vi "Experiment 20.vi"() -> ()   [LabVIEW 2026]
doc: "Experiment 20\nThis experiment is like Experiment 18 but uses while loops instead of for loops."
uses:
  <vilib>/AdvancedString/1D String Array to Delimited String (string).vi
  <vilib>/Analysis/baseanly.llb/Mean (DBL).vi
  <vilib>/Analysis/NI_AALBase.lvlib
panel:
  out "No. Of Iterations As Block Of Text (easy to copy into Excel)":string
  out "No. Of Iterations Executed - Loop 8":i32
  out "Output - Loop 8":dbl[](array[numeric]) format="%.3f"
  out "No. Of Iterations Executed - Loop 7":i32
  out "Output - Loop 7":dbl[](array[numeric]) format="%.3f"
  out "No. Of Iterations Executed - Loop 6":i32
  out "Output - Loop 6":dbl[](array[numeric]) format="%.3f"
  out "No. Of Iterations Executed - Loop 5":i32
  out "Output - Loop 5":dbl[](array[numeric]) format="%.3f"
  out "No. Of Iterations Executed - Loop 4":i32
  out "Output - Loop 4":dbl[](array[numeric]) format="%.3f"
  out "No. Of Iterations Executed - Loop 3":i32
  out "Output - Loop 3":dbl[](array[numeric]) format="%.3f"
  out "Avg. No. Of Iterations Executed - All Loops":dbl format="%.1f"
  out "No. Of Iterations Executed - Loop 2":i32
  out "Output - Loop 2":dbl[](array[numeric]) format="%.3f"
  out "No. Of Iterations Executed - Loop 1":i32
  out "Output - Loop 1":dbl[](array[numeric]) format="%.3f"
  out "Stop VI?":bool
  # "Experiment 20"
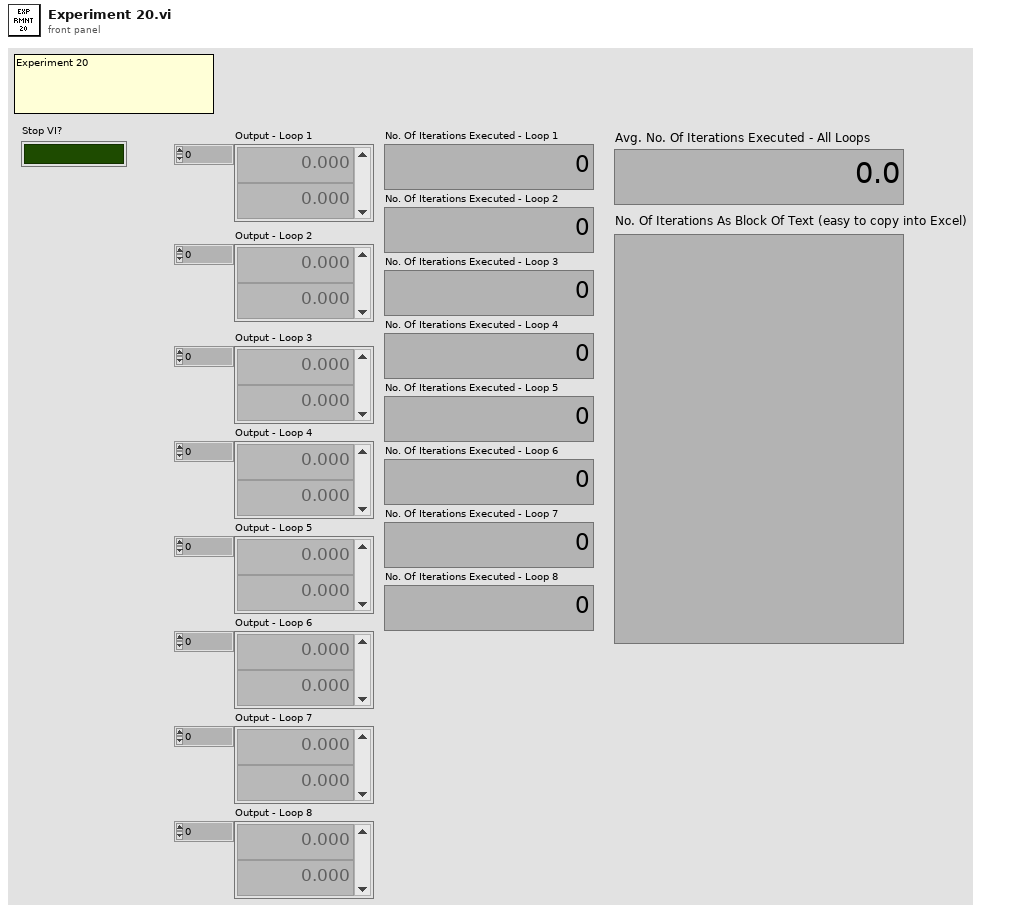
[diagram p1: front panel]
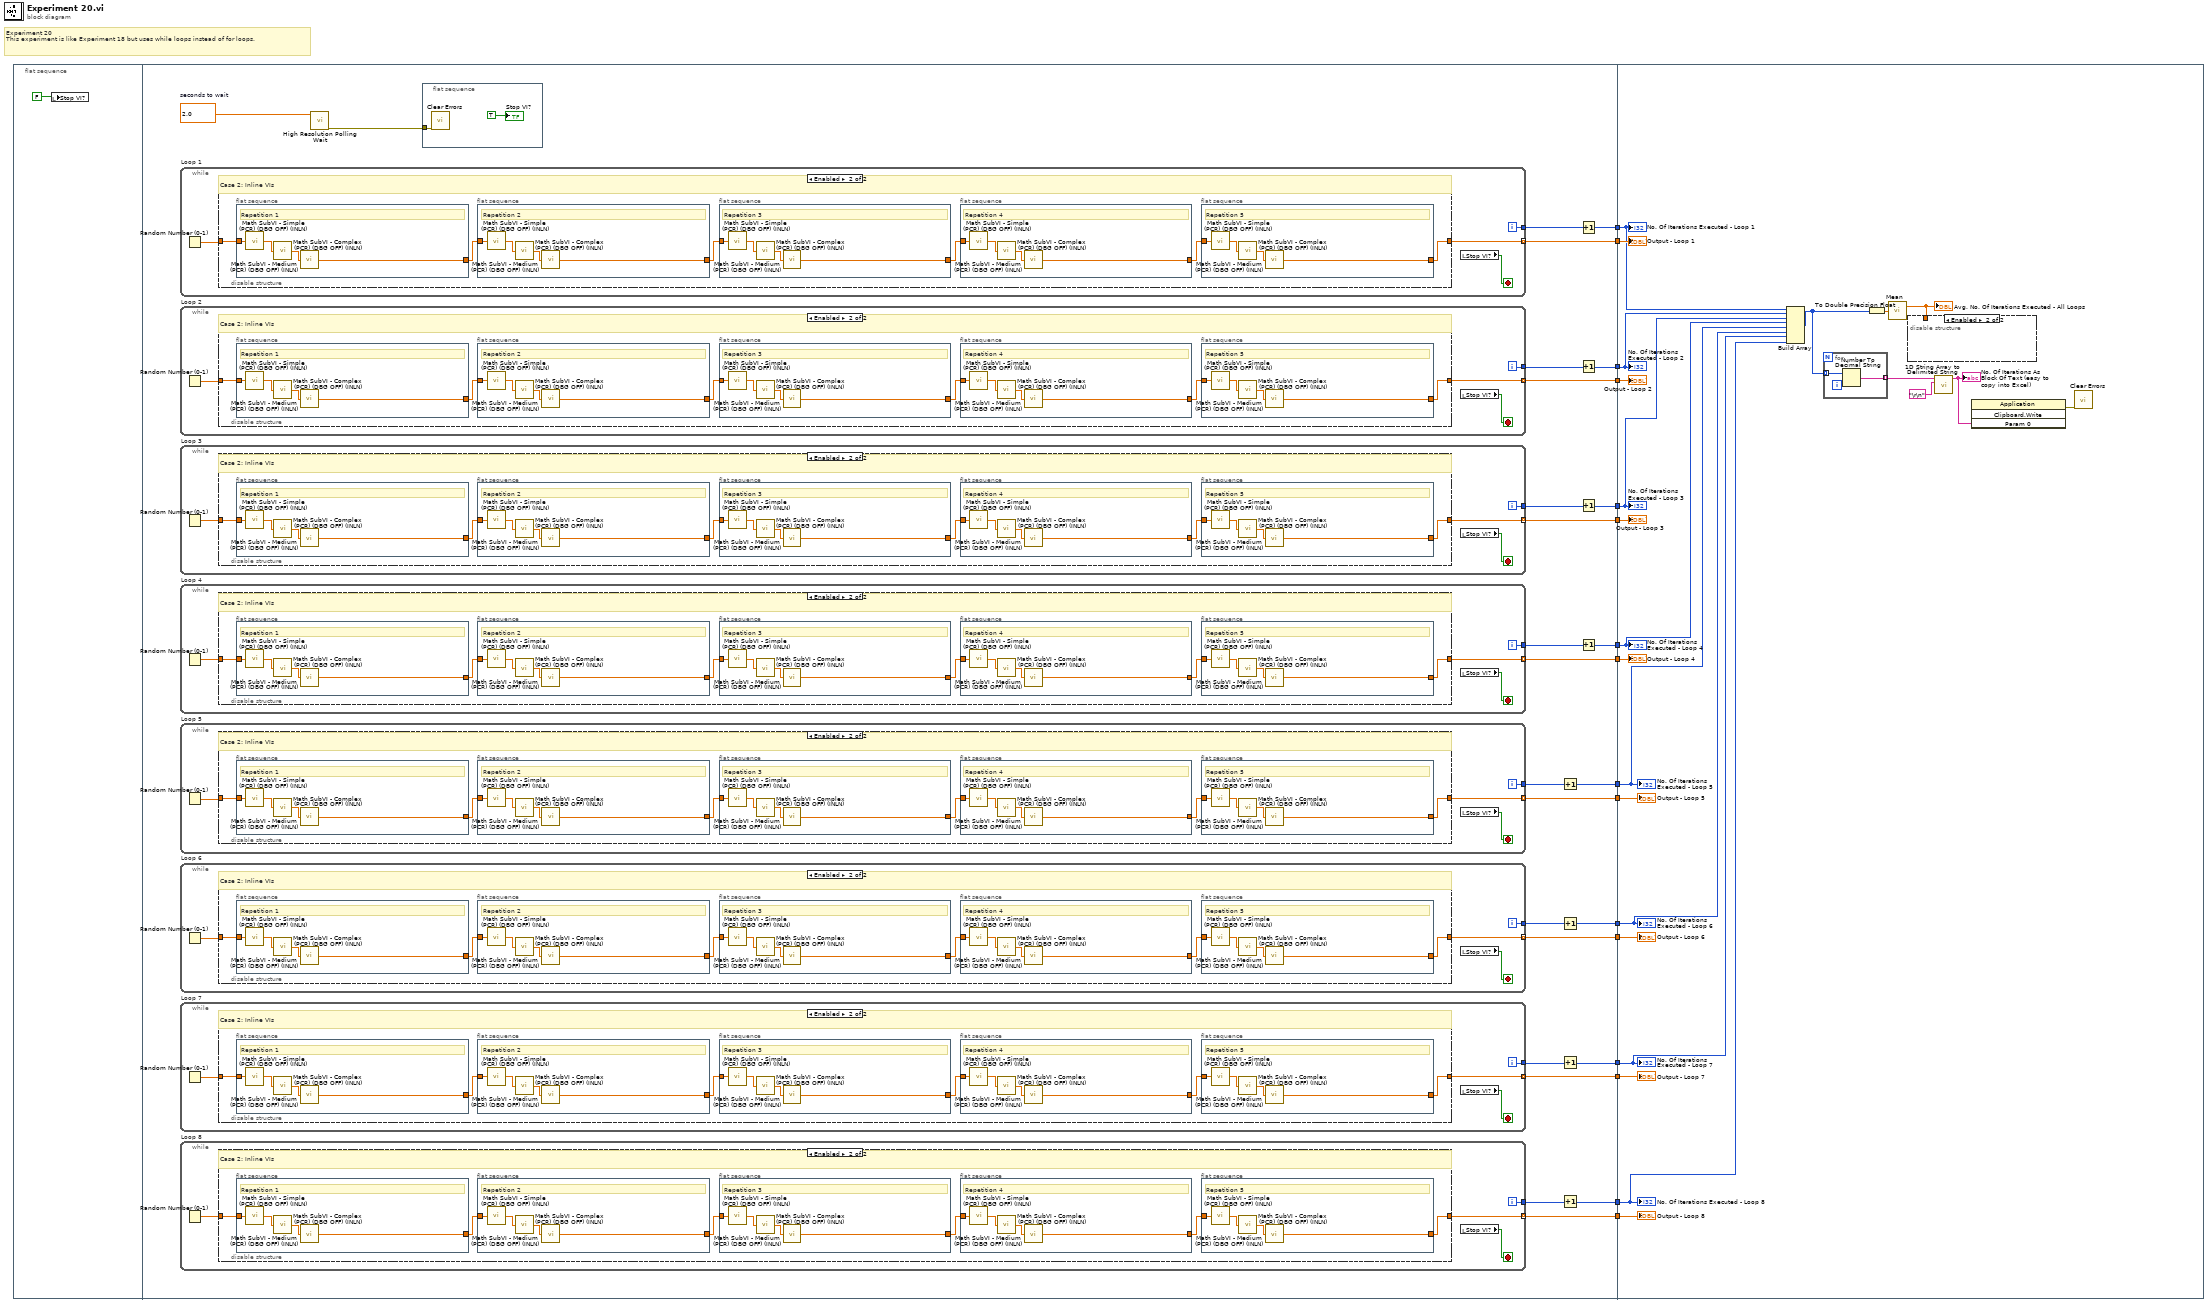
[diagram p0: block diagram]
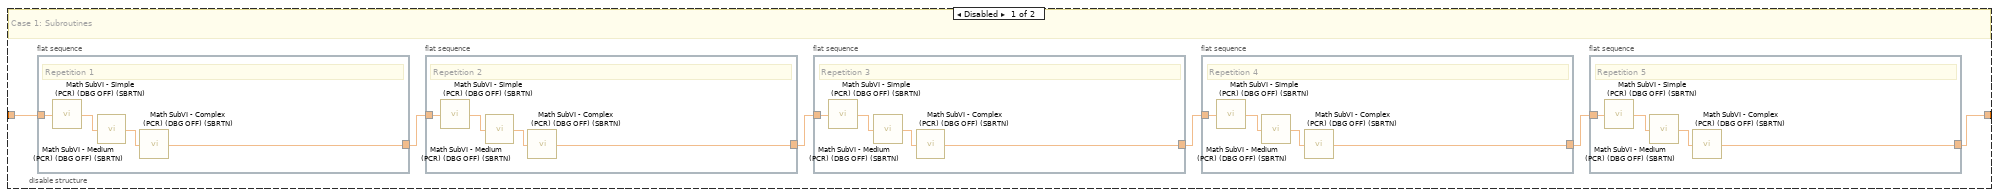
[diagram p2: hidden frame]
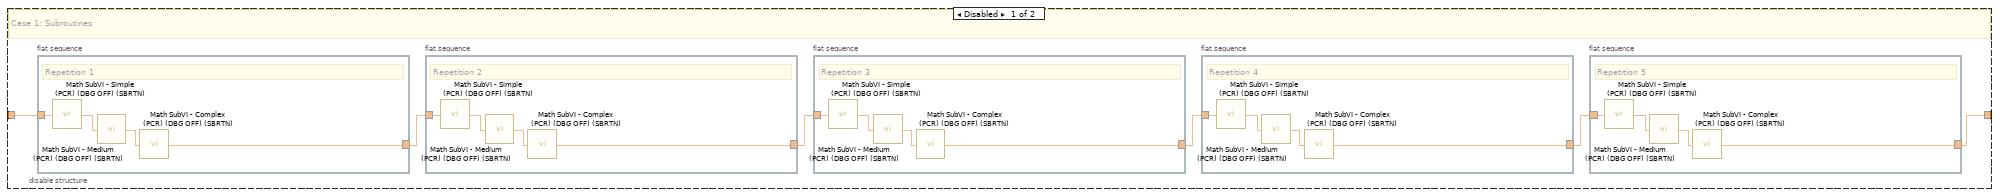
[diagram p3: hidden frame]
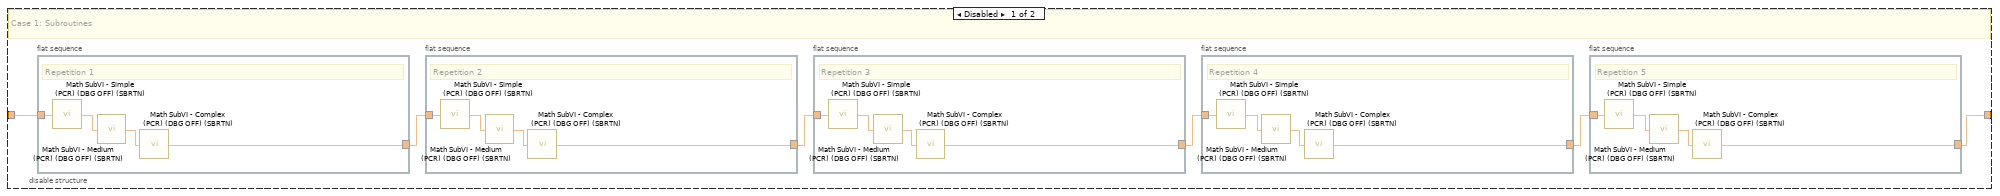
[diagram p4: hidden frame]
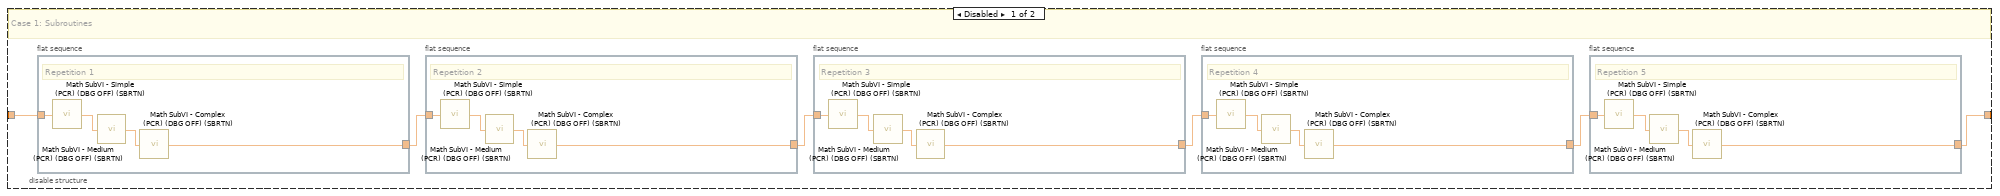
[diagram p5: hidden frame]
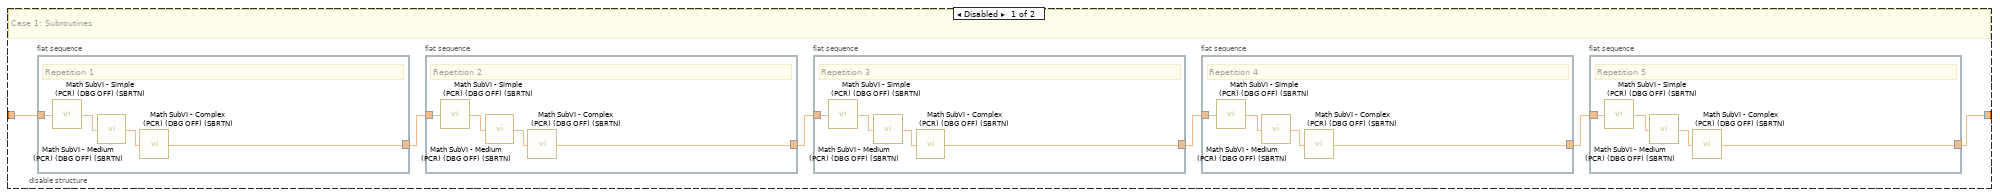
[diagram p6: hidden frame]
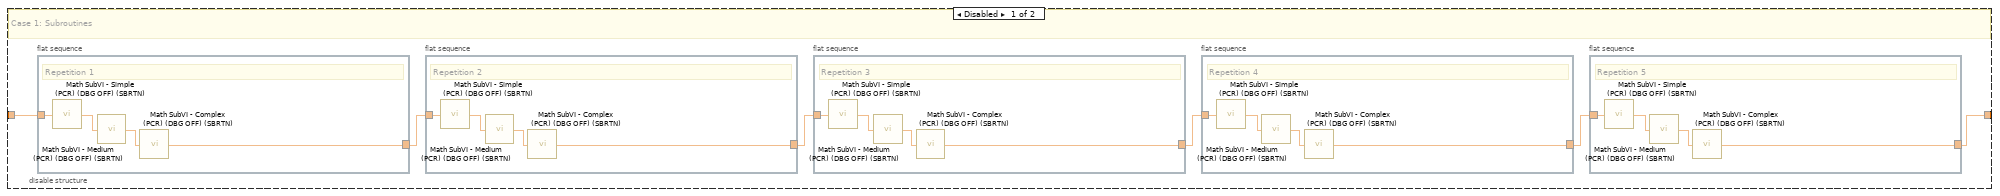
[diagram p7: hidden frame]
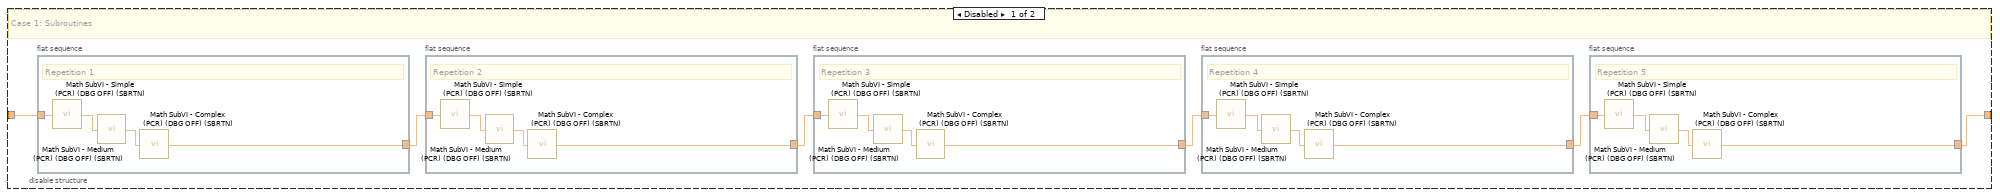
[diagram p8: hidden frame]
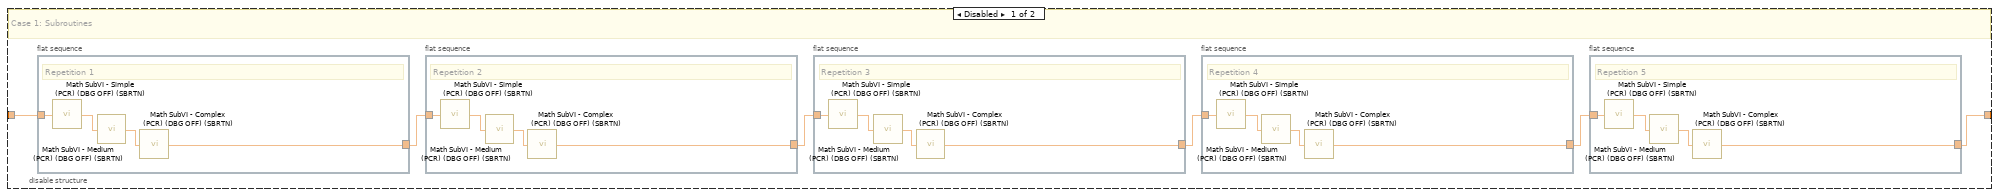
[diagram p9: hidden frame]
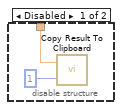
[diagram p10: hidden frame]
diagram:
  # "Experiment 20\nThis experiment is like Experiment 18 but uses while loops instead of for loops."
  n1 = flat-sequence {
    tunnel: [w41] -> w16
    tunnel: [w39] -> w15
    tunnel: [w38] -> w14
    tunnel: [w31] -> w13
    tunnel: [w37] -> w12
    tunnel: [w29] -> w11
    tunnel: [w27] -> w10
    tunnel: [w36] -> w9
    tunnel: [w25] -> w8
    tunnel: [w35] -> w7
    tunnel: [w23] -> w6
    tunnel: [w32] -> w5
    tunnel: [w21] -> w4
    tunnel: [w33] -> w3
    tunnel: [w18] -> w2
    tunnel: [w34] -> w1
    tunnel: w16 -> [w516]
    tunnel: w15 -> [w514]
    tunnel: w14 -> [w513]
    tunnel: w13 -> [w515]
    tunnel: w12 -> [w509]
    tunnel: w11 -> [w511]
    tunnel: w10 -> [w510]
    tunnel: w9 -> [w508]
    tunnel: w8 -> [w506]
    tunnel: w7 -> [w502]
    tunnel: w6 -> [w505]
    tunnel: w5 -> [w501]
    tunnel: w4 -> [w504]
    tunnel: w3 -> [w500]
    tunnel: w2 -> [w503]
    tunnel: w1 -> [w499]
    frame #0 {
      n2 = local write "Stop VI?"(FALSE) -> ()
    }
    frame #1 {
      w43 = 2.0  # seconds to wait
      n3 = while "Loop 1" {
        tunnel: [w437] -> w41 mode=indexing
        tunnel: [w438] -> w40
        i -> [w438]
        stop <- w439 stop-if-true
        n4 = Random Number (0-1)() -> (number: 0 to 1=w436:dbl)
        n5 = disable-structure shown="Enabled" {
          disable-tunnel: w436 -> [w445 w471]
          disable-tunnel: [w444 w466] -> w437
          frame Disabled {
            # "Case 1: Subroutines"
            n6 = flat-sequence {
              tunnel: w445 -> [w465]
              tunnel: [w462] -> w440
              frame #0 {
                # "Repetition 1"
                n7 = call "Math SubVI - Simple (PCR) (DBG OFF) (SBRTN).vi"("Input"=w465) -> ("Output"=w463:dbl)
                n8 = call "Math SubVI - Medium (PCR) (DBG OFF) (SBRTN).vi"("Input"=w463) -> ("Output"=w464:dbl)
                n9 = call "Math SubVI - Complex (PCR) (DBG OFF) (SBRTN).vi"("Input"=w464) -> ("Output"=w462:dbl)
              }
            }
            n10 = flat-sequence {
              tunnel: w440 -> [w461]
              tunnel: [w458] -> w443
              frame #0 {
                # "Repetition 2"
                n11 = call "Math SubVI - Simple (PCR) (DBG OFF) (SBRTN).vi"("Input"=w461) -> ("Output"=w459:dbl)
                n12 = call "Math SubVI - Medium (PCR) (DBG OFF) (SBRTN).vi"("Input"=w459) -> ("Output"=w460:dbl)
                n13 = call "Math SubVI - Complex (PCR) (DBG OFF) (SBRTN).vi"("Input"=w460) -> ("Output"=w458:dbl)
              }
            }
            n14 = flat-sequence {
              tunnel: w443 -> [w457]
              tunnel: [w454] -> w442
              frame #0 {
                # "Repetition 3"
                n15 = call "Math SubVI - Simple (PCR) (DBG OFF) (SBRTN).vi"("Input"=w457) -> ("Output"=w455:dbl)
                n16 = call "Math SubVI - Medium (PCR) (DBG OFF) (SBRTN).vi"("Input"=w455) -> ("Output"=w456:dbl)
                n17 = call "Math SubVI - Complex (PCR) (DBG OFF) (SBRTN).vi"("Input"=w456) -> ("Output"=w454:dbl)
              }
            }
            n18 = flat-sequence {
              tunnel: w442 -> [w453]
              tunnel: [w450] -> w441
              frame #0 {
                # "Repetition 4"
                n19 = call "Math SubVI - Simple (PCR) (DBG OFF) (SBRTN).vi"("Input"=w453) -> ("Output"=w451:dbl)
                n20 = call "Math SubVI - Medium (PCR) (DBG OFF) (SBRTN).vi"("Input"=w451) -> ("Output"=w452:dbl)
                n21 = call "Math SubVI - Complex (PCR) (DBG OFF) (SBRTN).vi"("Input"=w452) -> ("Output"=w450:dbl)
              }
            }
            n22 = flat-sequence {
              tunnel: w441 -> [w449]
              tunnel: [w446] -> w444
              frame #0 {
                # "Repetition 5"
                n23 = call "Math SubVI - Simple (PCR) (DBG OFF) (SBRTN).vi"("Input"=w449) -> ("Output"=w447:dbl)
                n24 = call "Math SubVI - Medium (PCR) (DBG OFF) (SBRTN).vi"("Input"=w447) -> ("Output"=w448:dbl)
                n25 = call "Math SubVI - Complex (PCR) (DBG OFF) (SBRTN).vi"("Input"=w448) -> ("Output"=w446:dbl)
              }
            }
          }
          frame Enabled {
            # "Case 2: Inline VIs"
            n26 = flat-sequence {
              tunnel: w471 -> [w491]
              tunnel: [w488] -> w470
              frame #0 {
                # "Repetition 1"
                n27 = call "Math SubVI - Simple (PCR) (DBG OFF) (INLN).vi"("Input"=w491) -> ("Output"=w489:dbl)
                n28 = call "Math SubVI - Medium (PCR) (DBG OFF) (INLN).vi"("Input"=w489) -> ("Output"=w490:dbl)
                n29 = call "Math SubVI - Complex (PCR) (DBG OFF) (INLN).vi"("Input"=w490) -> ("Output"=w488:dbl)
              }
            }
            n30 = flat-sequence {
              tunnel: w470 -> [w487]
              tunnel: [w484] -> w469
              frame #0 {
                # "Repetition 2"
                n31 = call "Math SubVI - Simple (PCR) (DBG OFF) (INLN).vi"("Input"=w487) -> ("Output"=w485:dbl)
                n32 = call "Math SubVI - Medium (PCR) (DBG OFF) (INLN).vi"("Input"=w485) -> ("Output"=w486:dbl)
                n33 = call "Math SubVI - Complex (PCR) (DBG OFF) (INLN).vi"("Input"=w486) -> ("Output"=w484:dbl)
              }
            }
            n34 = flat-sequence {
              tunnel: w469 -> [w483]
              tunnel: [w480] -> w468
              frame #0 {
                # "Repetition 3"
                n35 = call "Math SubVI - Simple (PCR) (DBG OFF) (INLN).vi"("Input"=w483) -> ("Output"=w481:dbl)
                n36 = call "Math SubVI - Medium (PCR) (DBG OFF) (INLN).vi"("Input"=w481) -> ("Output"=w482:dbl)
                n37 = call "Math SubVI - Complex (PCR) (DBG OFF) (INLN).vi"("Input"=w482) -> ("Output"=w480:dbl)
              }
            }
            n38 = flat-sequence {
              tunnel: w468 -> [w479]
              tunnel: [w476] -> w467
              frame #0 {
                # "Repetition 4"
                n39 = call "Math SubVI - Simple (PCR) (DBG OFF) (INLN).vi"("Input"=w479) -> ("Output"=w477:dbl)
                n40 = call "Math SubVI - Medium (PCR) (DBG OFF) (INLN).vi"("Input"=w477) -> ("Output"=w478:dbl)
                n41 = call "Math SubVI - Complex (PCR) (DBG OFF) (INLN).vi"("Input"=w478) -> ("Output"=w476:dbl)
              }
            }
            n42 = flat-sequence {
              tunnel: w467 -> [w475]
              tunnel: [w472] -> w466
              frame #0 {
                # "Repetition 5"
                n43 = call "Math SubVI - Simple (PCR) (DBG OFF) (INLN).vi"("Input"=w475) -> ("Output"=w473:dbl)
                n44 = call "Math SubVI - Medium (PCR) (DBG OFF) (INLN).vi"("Input"=w473) -> ("Output"=w474:dbl)
                n45 = call "Math SubVI - Complex (PCR) (DBG OFF) (INLN).vi"("Input"=w474) -> ("Output"=w472:dbl)
              }
            }
          }
        }
        n46 = local read "Stop VI?"() -> (w439:bool)
      }
      n47 = while "Loop 2" {
        tunnel: [w381] -> w31 mode=indexing
        tunnel: [w382] -> w30
        i -> [w382]
        stop <- w383 stop-if-true
        n48 = Random Number (0-1)() -> (number: 0 to 1=w380:dbl)
        n49 = disable-structure shown="Enabled" {
          disable-tunnel: w380 -> [w389 w415]
          disable-tunnel: [w388 w410] -> w381
          frame Disabled {
            # "Case 1: Subroutines"
            n50 = flat-sequence {
              tunnel: w389 -> [w409]
              tunnel: [w406] -> w384
              frame #0 {
                # "Repetition 1"
                n51 = call "Math SubVI - Simple (PCR) (DBG OFF) (SBRTN).vi"("Input"=w409) -> ("Output"=w407:dbl)
                n52 = call "Math SubVI - Medium (PCR) (DBG OFF) (SBRTN).vi"("Input"=w407) -> ("Output"=w408:dbl)
                n53 = call "Math SubVI - Complex (PCR) (DBG OFF) (SBRTN).vi"("Input"=w408) -> ("Output"=w406:dbl)
              }
            }
            n54 = flat-sequence {
              tunnel: w384 -> [w405]
              tunnel: [w402] -> w387
              frame #0 {
                # "Repetition 2"
                n55 = call "Math SubVI - Simple (PCR) (DBG OFF) (SBRTN).vi"("Input"=w405) -> ("Output"=w403:dbl)
                n56 = call "Math SubVI - Medium (PCR) (DBG OFF) (SBRTN).vi"("Input"=w403) -> ("Output"=w404:dbl)
                n57 = call "Math SubVI - Complex (PCR) (DBG OFF) (SBRTN).vi"("Input"=w404) -> ("Output"=w402:dbl)
              }
            }
            n58 = flat-sequence {
              tunnel: w387 -> [w401]
              tunnel: [w398] -> w386
              frame #0 {
                # "Repetition 3"
                n59 = call "Math SubVI - Simple (PCR) (DBG OFF) (SBRTN).vi"("Input"=w401) -> ("Output"=w399:dbl)
                n60 = call "Math SubVI - Medium (PCR) (DBG OFF) (SBRTN).vi"("Input"=w399) -> ("Output"=w400:dbl)
                n61 = call "Math SubVI - Complex (PCR) (DBG OFF) (SBRTN).vi"("Input"=w400) -> ("Output"=w398:dbl)
              }
            }
            n62 = flat-sequence {
              tunnel: w386 -> [w397]
              tunnel: [w394] -> w385
              frame #0 {
                # "Repetition 4"
                n63 = call "Math SubVI - Simple (PCR) (DBG OFF) (SBRTN).vi"("Input"=w397) -> ("Output"=w395:dbl)
                n64 = call "Math SubVI - Medium (PCR) (DBG OFF) (SBRTN).vi"("Input"=w395) -> ("Output"=w396:dbl)
                n65 = call "Math SubVI - Complex (PCR) (DBG OFF) (SBRTN).vi"("Input"=w396) -> ("Output"=w394:dbl)
              }
            }
            n66 = flat-sequence {
              tunnel: w385 -> [w393]
              tunnel: [w390] -> w388
              frame #0 {
                # "Repetition 5"
                n67 = call "Math SubVI - Simple (PCR) (DBG OFF) (SBRTN).vi"("Input"=w393) -> ("Output"=w391:dbl)
                n68 = call "Math SubVI - Medium (PCR) (DBG OFF) (SBRTN).vi"("Input"=w391) -> ("Output"=w392:dbl)
                n69 = call "Math SubVI - Complex (PCR) (DBG OFF) (SBRTN).vi"("Input"=w392) -> ("Output"=w390:dbl)
              }
            }
          }
          frame Enabled {
            # "Case 2: Inline VIs"
            n70 = flat-sequence {
              tunnel: w415 -> [w435]
              tunnel: [w432] -> w414
              frame #0 {
                # "Repetition 1"
                n71 = call "Math SubVI - Simple (PCR) (DBG OFF) (INLN).vi"("Input"=w435) -> ("Output"=w433:dbl)
                n72 = call "Math SubVI - Medium (PCR) (DBG OFF) (INLN).vi"("Input"=w433) -> ("Output"=w434:dbl)
                n73 = call "Math SubVI - Complex (PCR) (DBG OFF) (INLN).vi"("Input"=w434) -> ("Output"=w432:dbl)
              }
            }
            n74 = flat-sequence {
              tunnel: w414 -> [w431]
              tunnel: [w428] -> w413
              frame #0 {
                # "Repetition 2"
                n75 = call "Math SubVI - Simple (PCR) (DBG OFF) (INLN).vi"("Input"=w431) -> ("Output"=w429:dbl)
                n76 = call "Math SubVI - Medium (PCR) (DBG OFF) (INLN).vi"("Input"=w429) -> ("Output"=w430:dbl)
                n77 = call "Math SubVI - Complex (PCR) (DBG OFF) (INLN).vi"("Input"=w430) -> ("Output"=w428:dbl)
              }
            }
            n78 = flat-sequence {
              tunnel: w413 -> [w427]
              tunnel: [w424] -> w412
              frame #0 {
                # "Repetition 3"
                n79 = call "Math SubVI - Simple (PCR) (DBG OFF) (INLN).vi"("Input"=w427) -> ("Output"=w425:dbl)
                n80 = call "Math SubVI - Medium (PCR) (DBG OFF) (INLN).vi"("Input"=w425) -> ("Output"=w426:dbl)
                n81 = call "Math SubVI - Complex (PCR) (DBG OFF) (INLN).vi"("Input"=w426) -> ("Output"=w424:dbl)
              }
            }
            n82 = flat-sequence {
              tunnel: w412 -> [w423]
              tunnel: [w420] -> w411
              frame #0 {
                # "Repetition 4"
                n83 = call "Math SubVI - Simple (PCR) (DBG OFF) (INLN).vi"("Input"=w423) -> ("Output"=w421:dbl)
                n84 = call "Math SubVI - Medium (PCR) (DBG OFF) (INLN).vi"("Input"=w421) -> ("Output"=w422:dbl)
                n85 = call "Math SubVI - Complex (PCR) (DBG OFF) (INLN).vi"("Input"=w422) -> ("Output"=w420:dbl)
              }
            }
            n86 = flat-sequence {
              tunnel: w411 -> [w419]
              tunnel: [w416] -> w410
              frame #0 {
                # "Repetition 5"
                n87 = call "Math SubVI - Simple (PCR) (DBG OFF) (INLN).vi"("Input"=w419) -> ("Output"=w417:dbl)
                n88 = call "Math SubVI - Medium (PCR) (DBG OFF) (INLN).vi"("Input"=w417) -> ("Output"=w418:dbl)
                n89 = call "Math SubVI - Complex (PCR) (DBG OFF) (INLN).vi"("Input"=w418) -> ("Output"=w416:dbl)
              }
            }
          }
        }
        n90 = local read "Stop VI?"() -> (w383:bool)
      }
      n91 = while "Loop 3" {
        tunnel: [w325] -> w29 mode=indexing
        tunnel: [w326] -> w28
        i -> [w326]
        stop <- w327 stop-if-true
        n92 = Random Number (0-1)() -> (number: 0 to 1=w324:dbl)
        n93 = disable-structure shown="Enabled" {
          disable-tunnel: w324 -> [w333 w359]
          disable-tunnel: [w332 w354] -> w325
          frame Disabled {
            # "Case 1: Subroutines"
            n94 = flat-sequence {
              tunnel: w333 -> [w353]
              tunnel: [w350] -> w328
              frame #0 {
                # "Repetition 1"
                n95 = call "Math SubVI - Simple (PCR) (DBG OFF) (SBRTN).vi"("Input"=w353) -> ("Output"=w351:dbl)
                n96 = call "Math SubVI - Medium (PCR) (DBG OFF) (SBRTN).vi"("Input"=w351) -> ("Output"=w352:dbl)
                n97 = call "Math SubVI - Complex (PCR) (DBG OFF) (SBRTN).vi"("Input"=w352) -> ("Output"=w350:dbl)
              }
            }
            n98 = flat-sequence {
              tunnel: w328 -> [w349]
              tunnel: [w346] -> w331
              frame #0 {
                # "Repetition 2"
                n99 = call "Math SubVI - Simple (PCR) (DBG OFF) (SBRTN).vi"("Input"=w349) -> ("Output"=w347:dbl)
                n100 = call "Math SubVI - Medium (PCR) (DBG OFF) (SBRTN).vi"("Input"=w347) -> ("Output"=w348:dbl)
                n101 = call "Math SubVI - Complex (PCR) (DBG OFF) (SBRTN).vi"("Input"=w348) -> ("Output"=w346:dbl)
              }
            }
            n102 = flat-sequence {
              tunnel: w331 -> [w345]
              tunnel: [w342] -> w330
              frame #0 {
                # "Repetition 3"
                n103 = call "Math SubVI - Simple (PCR) (DBG OFF) (SBRTN).vi"("Input"=w345) -> ("Output"=w343:dbl)
                n104 = call "Math SubVI - Medium (PCR) (DBG OFF) (SBRTN).vi"("Input"=w343) -> ("Output"=w344:dbl)
                n105 = call "Math SubVI - Complex (PCR) (DBG OFF) (SBRTN).vi"("Input"=w344) -> ("Output"=w342:dbl)
              }
            }
            n106 = flat-sequence {
              tunnel: w330 -> [w341]
              tunnel: [w338] -> w329
              frame #0 {
                # "Repetition 4"
                n107 = call "Math SubVI - Simple (PCR) (DBG OFF) (SBRTN).vi"("Input"=w341) -> ("Output"=w339:dbl)
                n108 = call "Math SubVI - Medium (PCR) (DBG OFF) (SBRTN).vi"("Input"=w339) -> ("Output"=w340:dbl)
                n109 = call "Math SubVI - Complex (PCR) (DBG OFF) (SBRTN).vi"("Input"=w340) -> ("Output"=w338:dbl)
              }
            }
            n110 = flat-sequence {
              tunnel: w329 -> [w337]
              tunnel: [w334] -> w332
              frame #0 {
                # "Repetition 5"
                n111 = call "Math SubVI - Simple (PCR) (DBG OFF) (SBRTN).vi"("Input"=w337) -> ("Output"=w335:dbl)
                n112 = call "Math SubVI - Medium (PCR) (DBG OFF) (SBRTN).vi"("Input"=w335) -> ("Output"=w336:dbl)
                n113 = call "Math SubVI - Complex (PCR) (DBG OFF) (SBRTN).vi"("Input"=w336) -> ("Output"=w334:dbl)
              }
            }
          }
          frame Enabled {
            # "Case 2: Inline VIs"
            n114 = flat-sequence {
              tunnel: w359 -> [w379]
              tunnel: [w376] -> w358
              frame #0 {
                # "Repetition 1"
                n115 = call "Math SubVI - Simple (PCR) (DBG OFF) (INLN).vi"("Input"=w379) -> ("Output"=w377:dbl)
                n116 = call "Math SubVI - Medium (PCR) (DBG OFF) (INLN).vi"("Input"=w377) -> ("Output"=w378:dbl)
                n117 = call "Math SubVI - Complex (PCR) (DBG OFF) (INLN).vi"("Input"=w378) -> ("Output"=w376:dbl)
              }
            }
            n118 = flat-sequence {
              tunnel: w358 -> [w375]
              tunnel: [w372] -> w357
              frame #0 {
                # "Repetition 2"
                n119 = call "Math SubVI - Simple (PCR) (DBG OFF) (INLN).vi"("Input"=w375) -> ("Output"=w373:dbl)
                n120 = call "Math SubVI - Medium (PCR) (DBG OFF) (INLN).vi"("Input"=w373) -> ("Output"=w374:dbl)
                n121 = call "Math SubVI - Complex (PCR) (DBG OFF) (INLN).vi"("Input"=w374) -> ("Output"=w372:dbl)
              }
            }
            n122 = flat-sequence {
              tunnel: w357 -> [w371]
              tunnel: [w368] -> w356
              frame #0 {
                # "Repetition 3"
                n123 = call "Math SubVI - Simple (PCR) (DBG OFF) (INLN).vi"("Input"=w371) -> ("Output"=w369:dbl)
                n124 = call "Math SubVI - Medium (PCR) (DBG OFF) (INLN).vi"("Input"=w369) -> ("Output"=w370:dbl)
                n125 = call "Math SubVI - Complex (PCR) (DBG OFF) (INLN).vi"("Input"=w370) -> ("Output"=w368:dbl)
              }
            }
            n126 = flat-sequence {
              tunnel: w356 -> [w367]
              tunnel: [w364] -> w355
              frame #0 {
                # "Repetition 4"
                n127 = call "Math SubVI - Simple (PCR) (DBG OFF) (INLN).vi"("Input"=w367) -> ("Output"=w365:dbl)
                n128 = call "Math SubVI - Medium (PCR) (DBG OFF) (INLN).vi"("Input"=w365) -> ("Output"=w366:dbl)
                n129 = call "Math SubVI - Complex (PCR) (DBG OFF) (INLN).vi"("Input"=w366) -> ("Output"=w364:dbl)
              }
            }
            n130 = flat-sequence {
              tunnel: w355 -> [w363]
              tunnel: [w360] -> w354
              frame #0 {
                # "Repetition 5"
                n131 = call "Math SubVI - Simple (PCR) (DBG OFF) (INLN).vi"("Input"=w363) -> ("Output"=w361:dbl)
                n132 = call "Math SubVI - Medium (PCR) (DBG OFF) (INLN).vi"("Input"=w361) -> ("Output"=w362:dbl)
                n133 = call "Math SubVI - Complex (PCR) (DBG OFF) (INLN).vi"("Input"=w362) -> ("Output"=w360:dbl)
              }
            }
          }
        }
        n134 = local read "Stop VI?"() -> (w327:bool)
      }
      n135 = while "Loop 4" {
        tunnel: [w269] -> w27 mode=indexing
        tunnel: [w270] -> w26
        i -> [w270]
        stop <- w271 stop-if-true
        n136 = Random Number (0-1)() -> (number: 0 to 1=w268:dbl)
        n137 = disable-structure shown="Enabled" {
          disable-tunnel: w268 -> [w277 w303]
          disable-tunnel: [w276 w298] -> w269
          frame Disabled {
            # "Case 1: Subroutines"
            n138 = flat-sequence {
              tunnel: w277 -> [w297]
              tunnel: [w294] -> w272
              frame #0 {
                # "Repetition 1"
                n139 = call "Math SubVI - Simple (PCR) (DBG OFF) (SBRTN).vi"("Input"=w297) -> ("Output"=w295:dbl)
                n140 = call "Math SubVI - Medium (PCR) (DBG OFF) (SBRTN).vi"("Input"=w295) -> ("Output"=w296:dbl)
                n141 = call "Math SubVI - Complex (PCR) (DBG OFF) (SBRTN).vi"("Input"=w296) -> ("Output"=w294:dbl)
              }
            }
            n142 = flat-sequence {
              tunnel: w272 -> [w293]
              tunnel: [w290] -> w275
              frame #0 {
                # "Repetition 2"
                n143 = call "Math SubVI - Simple (PCR) (DBG OFF) (SBRTN).vi"("Input"=w293) -> ("Output"=w291:dbl)
                n144 = call "Math SubVI - Medium (PCR) (DBG OFF) (SBRTN).vi"("Input"=w291) -> ("Output"=w292:dbl)
                n145 = call "Math SubVI - Complex (PCR) (DBG OFF) (SBRTN).vi"("Input"=w292) -> ("Output"=w290:dbl)
              }
            }
            n146 = flat-sequence {
              tunnel: w275 -> [w289]
              tunnel: [w286] -> w274
              frame #0 {
                # "Repetition 3"
                n147 = call "Math SubVI - Simple (PCR) (DBG OFF) (SBRTN).vi"("Input"=w289) -> ("Output"=w287:dbl)
                n148 = call "Math SubVI - Medium (PCR) (DBG OFF) (SBRTN).vi"("Input"=w287) -> ("Output"=w288:dbl)
                n149 = call "Math SubVI - Complex (PCR) (DBG OFF) (SBRTN).vi"("Input"=w288) -> ("Output"=w286:dbl)
              }
            }
            n150 = flat-sequence {
              tunnel: w274 -> [w285]
              tunnel: [w282] -> w273
              frame #0 {
                # "Repetition 4"
                n151 = call "Math SubVI - Simple (PCR) (DBG OFF) (SBRTN).vi"("Input"=w285) -> ("Output"=w283:dbl)
                n152 = call "Math SubVI - Medium (PCR) (DBG OFF) (SBRTN).vi"("Input"=w283) -> ("Output"=w284:dbl)
                n153 = call "Math SubVI - Complex (PCR) (DBG OFF) (SBRTN).vi"("Input"=w284) -> ("Output"=w282:dbl)
              }
            }
            n154 = flat-sequence {
              tunnel: w273 -> [w281]
              tunnel: [w278] -> w276
              frame #0 {
                # "Repetition 5"
                n155 = call "Math SubVI - Simple (PCR) (DBG OFF) (SBRTN).vi"("Input"=w281) -> ("Output"=w279:dbl)
                n156 = call "Math SubVI - Medium (PCR) (DBG OFF) (SBRTN).vi"("Input"=w279) -> ("Output"=w280:dbl)
                n157 = call "Math SubVI - Complex (PCR) (DBG OFF) (SBRTN).vi"("Input"=w280) -> ("Output"=w278:dbl)
              }
            }
          }
          frame Enabled {
            # "Case 2: Inline VIs"
            n158 = flat-sequence {
              tunnel: w303 -> [w323]
              tunnel: [w320] -> w302
              frame #0 {
                # "Repetition 1"
                n159 = call "Math SubVI - Simple (PCR) (DBG OFF) (INLN).vi"("Input"=w323) -> ("Output"=w321:dbl)
                n160 = call "Math SubVI - Medium (PCR) (DBG OFF) (INLN).vi"("Input"=w321) -> ("Output"=w322:dbl)
                n161 = call "Math SubVI - Complex (PCR) (DBG OFF) (INLN).vi"("Input"=w322) -> ("Output"=w320:dbl)
              }
            }
            n162 = flat-sequence {
              tunnel: w302 -> [w319]
              tunnel: [w316] -> w301
              frame #0 {
                # "Repetition 2"
                n163 = call "Math SubVI - Simple (PCR) (DBG OFF) (INLN).vi"("Input"=w319) -> ("Output"=w317:dbl)
                n164 = call "Math SubVI - Medium (PCR) (DBG OFF) (INLN).vi"("Input"=w317) -> ("Output"=w318:dbl)
                n165 = call "Math SubVI - Complex (PCR) (DBG OFF) (INLN).vi"("Input"=w318) -> ("Output"=w316:dbl)
              }
            }
            n166 = flat-sequence {
              tunnel: w301 -> [w315]
              tunnel: [w312] -> w300
              frame #0 {
                # "Repetition 3"
                n167 = call "Math SubVI - Simple (PCR) (DBG OFF) (INLN).vi"("Input"=w315) -> ("Output"=w313:dbl)
                n168 = call "Math SubVI - Medium (PCR) (DBG OFF) (INLN).vi"("Input"=w313) -> ("Output"=w314:dbl)
                n169 = call "Math SubVI - Complex (PCR) (DBG OFF) (INLN).vi"("Input"=w314) -> ("Output"=w312:dbl)
              }
            }
            n170 = flat-sequence {
              tunnel: w300 -> [w311]
              tunnel: [w308] -> w299
              frame #0 {
                # "Repetition 4"
                n171 = call "Math SubVI - Simple (PCR) (DBG OFF) (INLN).vi"("Input"=w311) -> ("Output"=w309:dbl)
                n172 = call "Math SubVI - Medium (PCR) (DBG OFF) (INLN).vi"("Input"=w309) -> ("Output"=w310:dbl)
                n173 = call "Math SubVI - Complex (PCR) (DBG OFF) (INLN).vi"("Input"=w310) -> ("Output"=w308:dbl)
              }
            }
            n174 = flat-sequence {
              tunnel: w299 -> [w307]
              tunnel: [w304] -> w298
              frame #0 {
                # "Repetition 5"
                n175 = call "Math SubVI - Simple (PCR) (DBG OFF) (INLN).vi"("Input"=w307) -> ("Output"=w305:dbl)
                n176 = call "Math SubVI - Medium (PCR) (DBG OFF) (INLN).vi"("Input"=w305) -> ("Output"=w306:dbl)
                n177 = call "Math SubVI - Complex (PCR) (DBG OFF) (INLN).vi"("Input"=w306) -> ("Output"=w304:dbl)
              }
            }
          }
        }
        n178 = local read "Stop VI?"() -> (w271:bool)
      }
      n179 = while "Loop 5" {
        tunnel: [w213] -> w25 mode=indexing
        tunnel: [w214] -> w24
        i -> [w214]
        stop <- w215 stop-if-true
        n180 = Random Number (0-1)() -> (number: 0 to 1=w212:dbl)
        n181 = disable-structure shown="Enabled" {
          disable-tunnel: w212 -> [w221 w247]
          disable-tunnel: [w220 w242] -> w213
          frame Disabled {
            # "Case 1: Subroutines"
            n182 = flat-sequence {
              tunnel: w221 -> [w241]
              tunnel: [w238] -> w216
              frame #0 {
                # "Repetition 1"
                n183 = call "Math SubVI - Simple (PCR) (DBG OFF) (SBRTN).vi"("Input"=w241) -> ("Output"=w239:dbl)
                n184 = call "Math SubVI - Medium (PCR) (DBG OFF) (SBRTN).vi"("Input"=w239) -> ("Output"=w240:dbl)
                n185 = call "Math SubVI - Complex (PCR) (DBG OFF) (SBRTN).vi"("Input"=w240) -> ("Output"=w238:dbl)
              }
            }
            n186 = flat-sequence {
              tunnel: w216 -> [w237]
              tunnel: [w234] -> w219
              frame #0 {
                # "Repetition 2"
                n187 = call "Math SubVI - Simple (PCR) (DBG OFF) (SBRTN).vi"("Input"=w237) -> ("Output"=w235:dbl)
                n188 = call "Math SubVI - Medium (PCR) (DBG OFF) (SBRTN).vi"("Input"=w235) -> ("Output"=w236:dbl)
                n189 = call "Math SubVI - Complex (PCR) (DBG OFF) (SBRTN).vi"("Input"=w236) -> ("Output"=w234:dbl)
              }
            }
            n190 = flat-sequence {
              tunnel: w219 -> [w233]
              tunnel: [w230] -> w218
              frame #0 {
                # "Repetition 3"
                n191 = call "Math SubVI - Simple (PCR) (DBG OFF) (SBRTN).vi"("Input"=w233) -> ("Output"=w231:dbl)
                n192 = call "Math SubVI - Medium (PCR) (DBG OFF) (SBRTN).vi"("Input"=w231) -> ("Output"=w232:dbl)
                n193 = call "Math SubVI - Complex (PCR) (DBG OFF) (SBRTN).vi"("Input"=w232) -> ("Output"=w230:dbl)
              }
            }
            n194 = flat-sequence {
              tunnel: w218 -> [w229]
              tunnel: [w226] -> w217
              frame #0 {
                # "Repetition 4"
                n195 = call "Math SubVI - Simple (PCR) (DBG OFF) (SBRTN).vi"("Input"=w229) -> ("Output"=w227:dbl)
                n196 = call "Math SubVI - Medium (PCR) (DBG OFF) (SBRTN).vi"("Input"=w227) -> ("Output"=w228:dbl)
                n197 = call "Math SubVI - Complex (PCR) (DBG OFF) (SBRTN).vi"("Input"=w228) -> ("Output"=w226:dbl)
              }
            }
            n198 = flat-sequence {
              tunnel: w217 -> [w225]
              tunnel: [w222] -> w220
              frame #0 {
                # "Repetition 5"
                n199 = call "Math SubVI - Simple (PCR) (DBG OFF) (SBRTN).vi"("Input"=w225) -> ("Output"=w223:dbl)
                n200 = call "Math SubVI - Medium (PCR) (DBG OFF) (SBRTN).vi"("Input"=w223) -> ("Output"=w224:dbl)
                n201 = call "Math SubVI - Complex (PCR) (DBG OFF) (SBRTN).vi"("Input"=w224) -> ("Output"=w222:dbl)
              }
            }
          }
          frame Enabled {
            # "Case 2: Inline VIs"
            n202 = flat-sequence {
              tunnel: w247 -> [w267]
              tunnel: [w264] -> w246
              frame #0 {
                # "Repetition 1"
                n203 = call "Math SubVI - Simple (PCR) (DBG OFF) (INLN).vi"("Input"=w267) -> ("Output"=w265:dbl)
                n204 = call "Math SubVI - Medium (PCR) (DBG OFF) (INLN).vi"("Input"=w265) -> ("Output"=w266:dbl)
                n205 = call "Math SubVI - Complex (PCR) (DBG OFF) (INLN).vi"("Input"=w266) -> ("Output"=w264:dbl)
              }
            }
            n206 = flat-sequence {
              tunnel: w246 -> [w263]
              tunnel: [w260] -> w245
              frame #0 {
                # "Repetition 2"
                n207 = call "Math SubVI - Simple (PCR) (DBG OFF) (INLN).vi"("Input"=w263) -> ("Output"=w261:dbl)
                n208 = call "Math SubVI - Medium (PCR) (DBG OFF) (INLN).vi"("Input"=w261) -> ("Output"=w262:dbl)
                n209 = call "Math SubVI - Complex (PCR) (DBG OFF) (INLN).vi"("Input"=w262) -> ("Output"=w260:dbl)
              }
            }
            n210 = flat-sequence {
              tunnel: w245 -> [w259]
              tunnel: [w256] -> w244
              frame #0 {
                # "Repetition 3"
                n211 = call "Math SubVI - Simple (PCR) (DBG OFF) (INLN).vi"("Input"=w259) -> ("Output"=w257:dbl)
                n212 = call "Math SubVI - Medium (PCR) (DBG OFF) (INLN).vi"("Input"=w257) -> ("Output"=w258:dbl)
                n213 = call "Math SubVI - Complex (PCR) (DBG OFF) (INLN).vi"("Input"=w258) -> ("Output"=w256:dbl)
              }
            }
            n214 = flat-sequence {
              tunnel: w244 -> [w255]
              tunnel: [w252] -> w243
              frame #0 {
                # "Repetition 4"
                n215 = call "Math SubVI - Simple (PCR) (DBG OFF) (INLN).vi"("Input"=w255) -> ("Output"=w253:dbl)
                n216 = call "Math SubVI - Medium (PCR) (DBG OFF) (INLN).vi"("Input"=w253) -> ("Output"=w254:dbl)
                n217 = call "Math SubVI - Complex (PCR) (DBG OFF) (INLN).vi"("Input"=w254) -> ("Output"=w252:dbl)
              }
            }
            n218 = flat-sequence {
              tunnel: w243 -> [w251]
              tunnel: [w248] -> w242
              frame #0 {
                # "Repetition 5"
                n219 = call "Math SubVI - Simple (PCR) (DBG OFF) (INLN).vi"("Input"=w251) -> ("Output"=w249:dbl)
                n220 = call "Math SubVI - Medium (PCR) (DBG OFF) (INLN).vi"("Input"=w249) -> ("Output"=w250:dbl)
                n221 = call "Math SubVI - Complex (PCR) (DBG OFF) (INLN).vi"("Input"=w250) -> ("Output"=w248:dbl)
              }
            }
          }
        }
        n222 = local read "Stop VI?"() -> (w215:bool)
      }
      n223 = while "Loop 6" {
        tunnel: [w157] -> w23 mode=indexing
        tunnel: [w158] -> w22
        i -> [w158]
        stop <- w159 stop-if-true
        n224 = Random Number (0-1)() -> (number: 0 to 1=w156:dbl)
        n225 = disable-structure shown="Enabled" {
          disable-tunnel: w156 -> [w165 w191]
          disable-tunnel: [w164 w186] -> w157
          frame Disabled {
            # "Case 1: Subroutines"
            n226 = flat-sequence {
              tunnel: w165 -> [w185]
              tunnel: [w182] -> w160
              frame #0 {
                # "Repetition 1"
                n227 = call "Math SubVI - Simple (PCR) (DBG OFF) (SBRTN).vi"("Input"=w185) -> ("Output"=w183:dbl)
                n228 = call "Math SubVI - Medium (PCR) (DBG OFF) (SBRTN).vi"("Input"=w183) -> ("Output"=w184:dbl)
                n229 = call "Math SubVI - Complex (PCR) (DBG OFF) (SBRTN).vi"("Input"=w184) -> ("Output"=w182:dbl)
              }
            }
            n230 = flat-sequence {
              tunnel: w160 -> [w181]
              tunnel: [w178] -> w163
              frame #0 {
                # "Repetition 2"
                n231 = call "Math SubVI - Simple (PCR) (DBG OFF) (SBRTN).vi"("Input"=w181) -> ("Output"=w179:dbl)
                n232 = call "Math SubVI - Medium (PCR) (DBG OFF) (SBRTN).vi"("Input"=w179) -> ("Output"=w180:dbl)
                n233 = call "Math SubVI - Complex (PCR) (DBG OFF) (SBRTN).vi"("Input"=w180) -> ("Output"=w178:dbl)
              }
            }
            n234 = flat-sequence {
              tunnel: w163 -> [w177]
              tunnel: [w174] -> w162
              frame #0 {
                # "Repetition 3"
                n235 = call "Math SubVI - Simple (PCR) (DBG OFF) (SBRTN).vi"("Input"=w177) -> ("Output"=w175:dbl)
                n236 = call "Math SubVI - Medium (PCR) (DBG OFF) (SBRTN).vi"("Input"=w175) -> ("Output"=w176:dbl)
                n237 = call "Math SubVI - Complex (PCR) (DBG OFF) (SBRTN).vi"("Input"=w176) -> ("Output"=w174:dbl)
              }
            }
            n238 = flat-sequence {
              tunnel: w162 -> [w173]
              tunnel: [w170] -> w161
              frame #0 {
                # "Repetition 4"
                n239 = call "Math SubVI - Simple (PCR) (DBG OFF) (SBRTN).vi"("Input"=w173) -> ("Output"=w171:dbl)
                n240 = call "Math SubVI - Medium (PCR) (DBG OFF) (SBRTN).vi"("Input"=w171) -> ("Output"=w172:dbl)
                n241 = call "Math SubVI - Complex (PCR) (DBG OFF) (SBRTN).vi"("Input"=w172) -> ("Output"=w170:dbl)
              }
            }
            n242 = flat-sequence {
              tunnel: w161 -> [w169]
              tunnel: [w166] -> w164
              frame #0 {
                # "Repetition 5"
                n243 = call "Math SubVI - Simple (PCR) (DBG OFF) (SBRTN).vi"("Input"=w169) -> ("Output"=w167:dbl)
                n244 = call "Math SubVI - Medium (PCR) (DBG OFF) (SBRTN).vi"("Input"=w167) -> ("Output"=w168:dbl)
                n245 = call "Math SubVI - Complex (PCR) (DBG OFF) (SBRTN).vi"("Input"=w168) -> ("Output"=w166:dbl)
              }
            }
          }
          frame Enabled {
            # "Case 2: Inline VIs"
            n246 = flat-sequence {
              tunnel: w191 -> [w211]
              tunnel: [w208] -> w190
              frame #0 {
                # "Repetition 1"
                n247 = call "Math SubVI - Simple (PCR) (DBG OFF) (INLN).vi"("Input"=w211) -> ("Output"=w209:dbl)
                n248 = call "Math SubVI - Medium (PCR) (DBG OFF) (INLN).vi"("Input"=w209) -> ("Output"=w210:dbl)
                n249 = call "Math SubVI - Complex (PCR) (DBG OFF) (INLN).vi"("Input"=w210) -> ("Output"=w208:dbl)
              }
            }
            n250 = flat-sequence {
              tunnel: w190 -> [w207]
              tunnel: [w204] -> w189
              frame #0 {
                # "Repetition 2"
                n251 = call "Math SubVI - Simple (PCR) (DBG OFF) (INLN).vi"("Input"=w207) -> ("Output"=w205:dbl)
                n252 = call "Math SubVI - Medium (PCR) (DBG OFF) (INLN).vi"("Input"=w205) -> ("Output"=w206:dbl)
                n253 = call "Math SubVI - Complex (PCR) (DBG OFF) (INLN).vi"("Input"=w206) -> ("Output"=w204:dbl)
              }
            }
            n254 = flat-sequence {
              tunnel: w189 -> [w203]
              tunnel: [w200] -> w188
              frame #0 {
                # "Repetition 3"
                n255 = call "Math SubVI - Simple (PCR) (DBG OFF) (INLN).vi"("Input"=w203) -> ("Output"=w201:dbl)
                n256 = call "Math SubVI - Medium (PCR) (DBG OFF) (INLN).vi"("Input"=w201) -> ("Output"=w202:dbl)
                n257 = call "Math SubVI - Complex (PCR) (DBG OFF) (INLN).vi"("Input"=w202) -> ("Output"=w200:dbl)
              }
            }
            n258 = flat-sequence {
              tunnel: w188 -> [w199]
              tunnel: [w196] -> w187
              frame #0 {
                # "Repetition 4"
                n259 = call "Math SubVI - Simple (PCR) (DBG OFF) (INLN).vi"("Input"=w199) -> ("Output"=w197:dbl)
                n260 = call "Math SubVI - Medium (PCR) (DBG OFF) (INLN).vi"("Input"=w197) -> ("Output"=w198:dbl)
                n261 = call "Math SubVI - Complex (PCR) (DBG OFF) (INLN).vi"("Input"=w198) -> ("Output"=w196:dbl)
              }
            }
            n262 = flat-sequence {
              tunnel: w187 -> [w195]
              tunnel: [w192] -> w186
              frame #0 {
                # "Repetition 5"
                n263 = call "Math SubVI - Simple (PCR) (DBG OFF) (INLN).vi"("Input"=w195) -> ("Output"=w193:dbl)
                n264 = call "Math SubVI - Medium (PCR) (DBG OFF) (INLN).vi"("Input"=w193) -> ("Output"=w194:dbl)
                n265 = call "Math SubVI - Complex (PCR) (DBG OFF) (INLN).vi"("Input"=w194) -> ("Output"=w192:dbl)
              }
            }
          }
        }
        n266 = local read "Stop VI?"() -> (w159:bool)
      }
      n267 = while "Loop 7" {
        tunnel: [w101] -> w21 mode=indexing
        tunnel: [w102] -> w20
        i -> [w102]
        stop <- w103 stop-if-true
        n268 = Random Number (0-1)() -> (number: 0 to 1=w100:dbl)
        n269 = disable-structure shown="Enabled" {
          disable-tunnel: w100 -> [w109 w135]
          disable-tunnel: [w108 w130] -> w101
          frame Disabled {
            # "Case 1: Subroutines"
            n270 = flat-sequence {
              tunnel: w109 -> [w129]
              tunnel: [w126] -> w104
              frame #0 {
                # "Repetition 1"
                n271 = call "Math SubVI - Simple (PCR) (DBG OFF) (SBRTN).vi"("Input"=w129) -> ("Output"=w127:dbl)
                n272 = call "Math SubVI - Medium (PCR) (DBG OFF) (SBRTN).vi"("Input"=w127) -> ("Output"=w128:dbl)
                n273 = call "Math SubVI - Complex (PCR) (DBG OFF) (SBRTN).vi"("Input"=w128) -> ("Output"=w126:dbl)
              }
            }
            n274 = flat-sequence {
              tunnel: w104 -> [w125]
              tunnel: [w122] -> w107
              frame #0 {
                # "Repetition 2"
                n275 = call "Math SubVI - Simple (PCR) (DBG OFF) (SBRTN).vi"("Input"=w125) -> ("Output"=w123:dbl)
                n276 = call "Math SubVI - Medium (PCR) (DBG OFF) (SBRTN).vi"("Input"=w123) -> ("Output"=w124:dbl)
                n277 = call "Math SubVI - Complex (PCR) (DBG OFF) (SBRTN).vi"("Input"=w124) -> ("Output"=w122:dbl)
              }
            }
            n278 = flat-sequence {
              tunnel: w107 -> [w121]
              tunnel: [w118] -> w106
              frame #0 {
                # "Repetition 3"
                n279 = call "Math SubVI - Simple (PCR) (DBG OFF) (SBRTN).vi"("Input"=w121) -> ("Output"=w119:dbl)
                n280 = call "Math SubVI - Medium (PCR) (DBG OFF) (SBRTN).vi"("Input"=w119) -> ("Output"=w120:dbl)
                n281 = call "Math SubVI - Complex (PCR) (DBG OFF) (SBRTN).vi"("Input"=w120) -> ("Output"=w118:dbl)
              }
            }
            n282 = flat-sequence {
              tunnel: w106 -> [w117]
              tunnel: [w114] -> w105
              frame #0 {
                # "Repetition 4"
                n283 = call "Math SubVI - Simple (PCR) (DBG OFF) (SBRTN).vi"("Input"=w117) -> ("Output"=w115:dbl)
                n284 = call "Math SubVI - Medium (PCR) (DBG OFF) (SBRTN).vi"("Input"=w115) -> ("Output"=w116:dbl)
                n285 = call "Math SubVI - Complex (PCR) (DBG OFF) (SBRTN).vi"("Input"=w116) -> ("Output"=w114:dbl)
              }
            }
            n286 = flat-sequence {
              tunnel: w105 -> [w113]
              tunnel: [w110] -> w108
              frame #0 {
                # "Repetition 5"
                n287 = call "Math SubVI - Simple (PCR) (DBG OFF) (SBRTN).vi"("Input"=w113) -> ("Output"=w111:dbl)
                n288 = call "Math SubVI - Medium (PCR) (DBG OFF) (SBRTN).vi"("Input"=w111) -> ("Output"=w112:dbl)
                n289 = call "Math SubVI - Complex (PCR) (DBG OFF) (SBRTN).vi"("Input"=w112) -> ("Output"=w110:dbl)
              }
            }
          }
          frame Enabled {
            # "Case 2: Inline VIs"
            n290 = flat-sequence {
              tunnel: w135 -> [w155]
              tunnel: [w152] -> w134
              frame #0 {
                # "Repetition 1"
                n291 = call "Math SubVI - Simple (PCR) (DBG OFF) (INLN).vi"("Input"=w155) -> ("Output"=w153:dbl)
                n292 = call "Math SubVI - Medium (PCR) (DBG OFF) (INLN).vi"("Input"=w153) -> ("Output"=w154:dbl)
                n293 = call "Math SubVI - Complex (PCR) (DBG OFF) (INLN).vi"("Input"=w154) -> ("Output"=w152:dbl)
              }
            }
            n294 = flat-sequence {
              tunnel: w134 -> [w151]
              tunnel: [w148] -> w133
              frame #0 {
                # "Repetition 2"
                n295 = call "Math SubVI - Simple (PCR) (DBG OFF) (INLN).vi"("Input"=w151) -> ("Output"=w149:dbl)
                n296 = call "Math SubVI - Medium (PCR) (DBG OFF) (INLN).vi"("Input"=w149) -> ("Output"=w150:dbl)
                n297 = call "Math SubVI - Complex (PCR) (DBG OFF) (INLN).vi"("Input"=w150) -> ("Output"=w148:dbl)
              }
            }
            n298 = flat-sequence {
              tunnel: w133 -> [w147]
              tunnel: [w144] -> w132
              frame #0 {
                # "Repetition 3"
                n299 = call "Math SubVI - Simple (PCR) (DBG OFF) (INLN).vi"("Input"=w147) -> ("Output"=w145:dbl)
                n300 = call "Math SubVI - Medium (PCR) (DBG OFF) (INLN).vi"("Input"=w145) -> ("Output"=w146:dbl)
                n301 = call "Math SubVI - Complex (PCR) (DBG OFF) (INLN).vi"("Input"=w146) -> ("Output"=w144:dbl)
              }
            }
            n302 = flat-sequence {
              tunnel: w132 -> [w143]
              tunnel: [w140] -> w131
              frame #0 {
                # "Repetition 4"
                n303 = call "Math SubVI - Simple (PCR) (DBG OFF) (INLN).vi"("Input"=w143) -> ("Output"=w141:dbl)
                n304 = call "Math SubVI - Medium (PCR) (DBG OFF) (INLN).vi"("Input"=w141) -> ("Output"=w142:dbl)
                n305 = call "Math SubVI - Complex (PCR) (DBG OFF) (INLN).vi"("Input"=w142) -> ("Output"=w140:dbl)
              }
            }
            n306 = flat-sequence {
              tunnel: w131 -> [w139]
              tunnel: [w136] -> w130
              frame #0 {
                # "Repetition 5"
                n307 = call "Math SubVI - Simple (PCR) (DBG OFF) (INLN).vi"("Input"=w139) -> ("Output"=w137:dbl)
                n308 = call "Math SubVI - Medium (PCR) (DBG OFF) (INLN).vi"("Input"=w137) -> ("Output"=w138:dbl)
                n309 = call "Math SubVI - Complex (PCR) (DBG OFF) (INLN).vi"("Input"=w138) -> ("Output"=w136:dbl)
              }
            }
          }
        }
        n310 = local read "Stop VI?"() -> (w103:bool)
      }
      n311 = while "Loop 8" {
        tunnel: [w45] -> w18 mode=indexing
        tunnel: [w46] -> w19
        i -> [w46]
        stop <- w47 stop-if-true
        n312 = Random Number (0-1)() -> (number: 0 to 1=w44:dbl)
        n313 = disable-structure shown="Enabled" {
          disable-tunnel: w44 -> [w53 w79]
          disable-tunnel: [w52 w74] -> w45
          frame Disabled {
            # "Case 1: Subroutines"
            n314 = flat-sequence {
              tunnel: w53 -> [w73]
              tunnel: [w70] -> w48
              frame #0 {
                # "Repetition 1"
                n315 = call "Math SubVI - Simple (PCR) (DBG OFF) (SBRTN).vi"("Input"=w73) -> ("Output"=w71:dbl)
                n316 = call "Math SubVI - Medium (PCR) (DBG OFF) (SBRTN).vi"("Input"=w71) -> ("Output"=w72:dbl)
                n317 = call "Math SubVI - Complex (PCR) (DBG OFF) (SBRTN).vi"("Input"=w72) -> ("Output"=w70:dbl)
              }
            }
            n318 = flat-sequence {
              tunnel: w48 -> [w69]
              tunnel: [w66] -> w51
              frame #0 {
                # "Repetition 2"
                n319 = call "Math SubVI - Simple (PCR) (DBG OFF) (SBRTN).vi"("Input"=w69) -> ("Output"=w67:dbl)
                n320 = call "Math SubVI - Medium (PCR) (DBG OFF) (SBRTN).vi"("Input"=w67) -> ("Output"=w68:dbl)
                n321 = call "Math SubVI - Complex (PCR) (DBG OFF) (SBRTN).vi"("Input"=w68) -> ("Output"=w66:dbl)
              }
            }
            n322 = flat-sequence {
              tunnel: w51 -> [w65]
              tunnel: [w62] -> w50
              frame #0 {
                # "Repetition 3"
                n323 = call "Math SubVI - Simple (PCR) (DBG OFF) (SBRTN).vi"("Input"=w65) -> ("Output"=w63:dbl)
                n324 = call "Math SubVI - Medium (PCR) (DBG OFF) (SBRTN).vi"("Input"=w63) -> ("Output"=w64:dbl)
                n325 = call "Math SubVI - Complex (PCR) (DBG OFF) (SBRTN).vi"("Input"=w64) -> ("Output"=w62:dbl)
              }
            }
            n326 = flat-sequence {
              tunnel: w50 -> [w61]
              tunnel: [w58] -> w49
              frame #0 {
                # "Repetition 4"
                n327 = call "Math SubVI - Simple (PCR) (DBG OFF) (SBRTN).vi"("Input"=w61) -> ("Output"=w59:dbl)
                n328 = call "Math SubVI - Medium (PCR) (DBG OFF) (SBRTN).vi"("Input"=w59) -> ("Output"=w60:dbl)
                n329 = call "Math SubVI - Complex (PCR) (DBG OFF) (SBRTN).vi"("Input"=w60) -> ("Output"=w58:dbl)
              }
            }
            n330 = flat-sequence {
              tunnel: w49 -> [w57]
              tunnel: [w54] -> w52
              frame #0 {
                # "Repetition 5"
                n331 = call "Math SubVI - Simple (PCR) (DBG OFF) (SBRTN).vi"("Input"=w57) -> ("Output"=w55:dbl)
                n332 = call "Math SubVI - Medium (PCR) (DBG OFF) (SBRTN).vi"("Input"=w55) -> ("Output"=w56:dbl)
                n333 = call "Math SubVI - Complex (PCR) (DBG OFF) (SBRTN).vi"("Input"=w56) -> ("Output"=w54:dbl)
              }
            }
          }
          frame Enabled {
            # "Case 2: Inline VIs"
            n334 = flat-sequence {
              tunnel: w79 -> [w99]
              tunnel: [w96] -> w78
              frame #0 {
                # "Repetition 1"
                n335 = call "Math SubVI - Simple (PCR) (DBG OFF) (INLN).vi"("Input"=w99) -> ("Output"=w97:dbl)
                n336 = call "Math SubVI - Medium (PCR) (DBG OFF) (INLN).vi"("Input"=w97) -> ("Output"=w98:dbl)
                n337 = call "Math SubVI - Complex (PCR) (DBG OFF) (INLN).vi"("Input"=w98) -> ("Output"=w96:dbl)
              }
            }
            n338 = flat-sequence {
              tunnel: w78 -> [w95]
              tunnel: [w92] -> w77
              frame #0 {
                # "Repetition 2"
                n339 = call "Math SubVI - Simple (PCR) (DBG OFF) (INLN).vi"("Input"=w95) -> ("Output"=w93:dbl)
                n340 = call "Math SubVI - Medium (PCR) (DBG OFF) (INLN).vi"("Input"=w93) -> ("Output"=w94:dbl)
                n341 = call "Math SubVI - Complex (PCR) (DBG OFF) (INLN).vi"("Input"=w94) -> ("Output"=w92:dbl)
              }
            }
            n342 = flat-sequence {
              tunnel: w77 -> [w91]
              tunnel: [w88] -> w76
              frame #0 {
                # "Repetition 3"
                n343 = call "Math SubVI - Simple (PCR) (DBG OFF) (INLN).vi"("Input"=w91) -> ("Output"=w89:dbl)
                n344 = call "Math SubVI - Medium (PCR) (DBG OFF) (INLN).vi"("Input"=w89) -> ("Output"=w90:dbl)
                n345 = call "Math SubVI - Complex (PCR) (DBG OFF) (INLN).vi"("Input"=w90) -> ("Output"=w88:dbl)
              }
            }
            n346 = flat-sequence {
              tunnel: w76 -> [w87]
              tunnel: [w84] -> w75
              frame #0 {
                # "Repetition 4"
                n347 = call "Math SubVI - Simple (PCR) (DBG OFF) (INLN).vi"("Input"=w87) -> ("Output"=w85:dbl)
                n348 = call "Math SubVI - Medium (PCR) (DBG OFF) (INLN).vi"("Input"=w85) -> ("Output"=w86:dbl)
                n349 = call "Math SubVI - Complex (PCR) (DBG OFF) (INLN).vi"("Input"=w86) -> ("Output"=w84:dbl)
              }
            }
            n350 = flat-sequence {
              tunnel: w75 -> [w83]
              tunnel: [w80] -> w74
              frame #0 {
                # "Repetition 5"
                n351 = call "Math SubVI - Simple (PCR) (DBG OFF) (INLN).vi"("Input"=w83) -> ("Output"=w81:dbl)
                n352 = call "Math SubVI - Medium (PCR) (DBG OFF) (INLN).vi"("Input"=w81) -> ("Output"=w82:dbl)
                n353 = call "Math SubVI - Complex (PCR) (DBG OFF) (INLN).vi"("Input"=w82) -> ("Output"=w80:dbl)
              }
            }
          }
        }
        n354 = local read "Stop VI?"() -> (w47:bool)
      }
      n355 = call <vilib>:"High Resolution Polling Wait.vi"("seconds to wait"=w43) -> ("error out"=w42:errorcluster)  [unwired: 10 in]
      n356 = flat-sequence {
        tunnel: w42 -> [w492]
        frame #0 {
          n357 = call <vilib>:"Clear Errors.vi"("error in (no error)"=w492) -> ()  [unwired: 5 in, 2 out]
          "Stop VI?" <- TRUE
        }
      }
      n358 = Increment(x=w24) -> (x+1=w35:i32)
      n359 = Increment(x=w22) -> (x+1=w32:i32)
      n360 = Increment(x=w20) -> (x+1=w33:i32)
      n361 = Increment(x=w19) -> (x+1=w34:i32)
      n362 = Increment(x=w40) -> (x+1=w39:i32)
      n363 = Increment(x=w30) -> (x+1=w38:i32)
      n364 = Increment(x=w28) -> (x+1=w37:i32)
      n365 = Increment(x=w26) -> (x+1=w36:i32)
    }
    frame #2 {
      n366 = Build Array(w514, w513, w509, w508, w502, w501, w500, w499) -> (w498:i32[])
      n367 = for {
        tunnel: w498 -> [w520] mode=indexing
        tunnel: [w519] -> w497 mode=indexing
        n368 = Number To Decimal String(number=w520) -> (decimal integer string=w519:string)  [unwired: 1 in]
      }
      n369 = To Double Precision Float(number=w498) -> (double precision float=w507:dbl[])
      n370 = call-poly <vilib>:"Mean.vi"("X"=w507) -> ("mean"=w512:dbl)  [unwired: 1 out]
      "Avg. No. Of Iterations Executed - All Loops" <- w512
      n371 = disable-structure shown="Enabled" {
        disable-tunnel: w512 -> [w518 _]
        frame Disabled {
          n372 = call "Copy Result To Clipboard.vi"("No. Of Decimal Places (6)"=u32 1, "Input"=w518) -> ()
        }
        frame Enabled {
        }
      }
      n373 = call-poly <vilib>:"1D String Array to Delimited String.vi"("delimiter"="\r\n", "string array"=w497) -> ("delimited string"=w494:string)  [unwired: 9 in]
      "No. Of Iterations As Block Of Text (easy to copy into Excel)" <- w494
      n374 = invoke class="Application" method="Clipboard.Write"("Param 0"=w494) -> (error out=w495:errorcluster)  [unwired: 3 in, 3 out]
      n375 = call <vilib>:"Clear Errors.vi"("error in (no error)"=w495) -> ()  [unwired: 5 in, 2 out]
      "No. Of Iterations Executed - Loop 1" <- w514
      "Output - Loop 1" <- w516
      "No. Of Iterations Executed - Loop 2" <- w513
      "Output - Loop 2" <- w515
      "No. Of Iterations Executed - Loop 3" <- w509
      "Output - Loop 3" <- w511
      "No. Of Iterations Executed - Loop 4" <- w508
      "Output - Loop 4" <- w510
      "No. Of Iterations Executed - Loop 5" <- w502
      "Output - Loop 5" <- w506
      "No. Of Iterations Executed - Loop 6" <- w501
      "Output - Loop 6" <- w505
      "No. Of Iterations Executed - Loop 7" <- w500
      "Output - Loop 7" <- w504
      "No. Of Iterations Executed - Loop 8" <- w499
      "Output - Loop 8" <- w503
    }
  }
